vi "Decode.vi"(3 "String":string) -> (0 "ON/OFF":bool, 1 "Relay Number":u8)   [LabVIEW 2020]
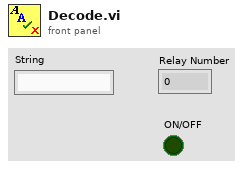
[diagram p1: front panel]
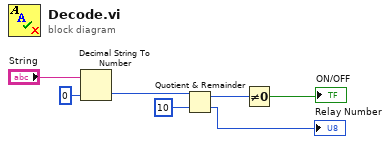
[diagram p0: block diagram]
diagram:
  n1 = Decimal String To Number(string="String", default (0L)=u8 0 ("default (0 I32)")) -> (number=w6:u8)  [unwired: 1 in, 1 out]
  n2 = Quotient & Remainder(x=w6, y=u8 10) -> (x-y*floor(x/y)=w5:u8, floor(x/y)=→"Relay Number":u8)
  n3 = Not Equal To 0?(x=w5) -> (x != 0?=→"ON/OFF":bool)
